vi "EMD8216 dll version read.vi"() -> (1 "sub_ver":u8, 2 "maj_ver":u8, 3 "error_code":u32)   [LabVIEW 2009, in "EMD8216_64.lvlib"]
doc: "EMD8216Status EMD8216_dll_version_read(u8 *maj_ver, u8 *sub_ver);"
uses:
  EMD8216_64.lvlib
  <userlib>/EMD8216_64/EMD8216_64.dll
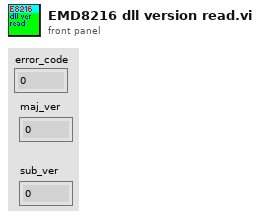
[diagram p1: front panel]
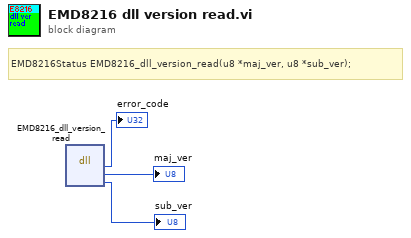
[diagram p0: block diagram]
diagram:
  # "EMD8216Status EMD8216_dll_version_read(u8 *maj_ver, u8 *sub_ver);"
  n1 = dll-call lib="C:/Program Files/National Instruments/LabVIEW 2017/user.lib/EMD8216_64/EMD8216_64.*" fn="EMD8216_dll_version_read"() -> ("error_code"=→"error_code":u32, "maj_ver"=→"maj_ver":u8, "sub_ver"=→"sub_ver":u8)  [unwired: 5 in, 2 out]
